vi "Fault Handling.vi"(8 "error in":errorcluster, 10 "FaultCode":i32, 11 "PostUUT in":refnum<class "PostUUT.lvclass">) -> (0 "error out":errorcluster, 3 "PostUUT out":refnum<class "PostUUT.lvclass">)   [LabVIEW 2021, in "PostUUT.lvclass"]
uses:
  PostUUT.lvclass
  PostUUT.lvclass/PostUUT.ctl
  OPC UA/OPC UA.lvclass
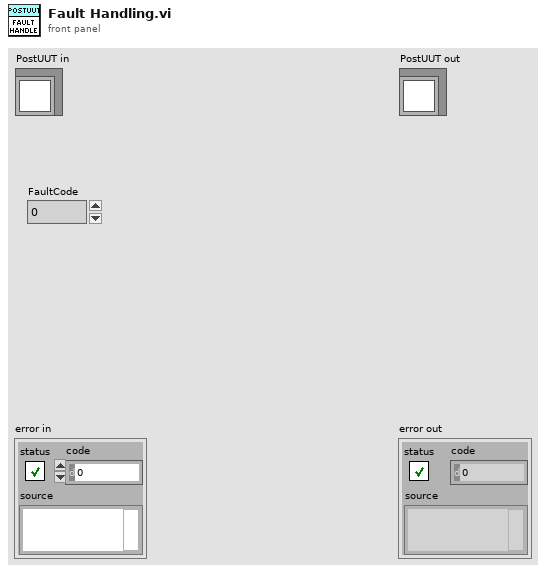
[diagram p1: front panel]
types:
  T1 = typedef "PostUUT.lvclass/Rx PostUUT.ctl" = cluster{"ResultsAck":bool, "Reset":bool, "Stop":bool, "FaultCode":u32}
  T2 = typedef "PostUUT.lvclass/Tx PostUUT.ctl" = cluster{"ResultsReady":bool, "Results":i32, "ElapsedTime":i32, "TimeCompleted":i32[], "Fault":bool, "Timeout":bool}
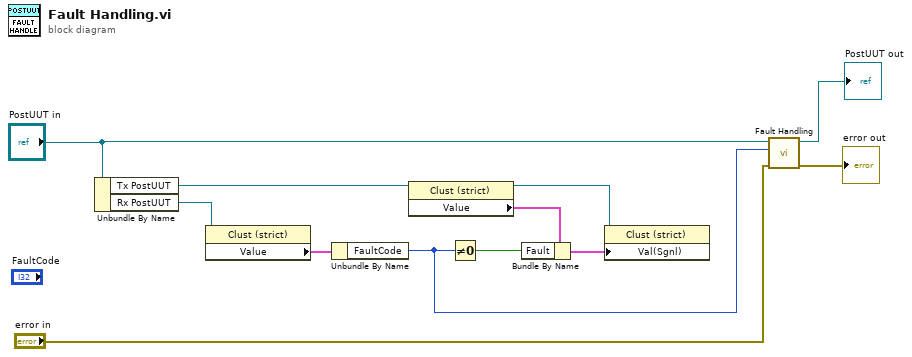
[diagram p0: block diagram]
diagram:
  n1 = Unbundle By Name("PostUUT in") -> ("Tx PostUUT"=w7:refnum<vi>, "Rx PostUUT"=w5:refnum<vi>)
  n2 = property class="Clust (strict)"(reference=w5) -> ("Value"=w6:T1)  [unwired: 1 in, 2 out]
  n3 = Unbundle By Name(w6) -> ("FaultCode"=w3:u32)
  n4 = property class="Clust (strict)"(reference=w7) -> (reference out=w10:refnum<vi>, "Value"=w8:T2)  [unwired: 1 in, 1 out]
  n5 = Not Equal To 0?(x=w3) -> (x != 0?=w2:bool)
  n6 = Bundle By Name(cluster=w8, "Fault"=w2) -> (w9:T2)
  n7 = property class="Clust (strict)"(reference=w10, "Val(Sgnl)"=w9) -> ()  [unwired: 1 in, 2 out]
  n8 = call-parent "Fault Handling.vi"("error in (no error)"="error in", "FaultCode"=w3, "OPC UA in"="PostUUT in") -> ("error out"=→"error out":errorcluster, "OPC UA out"=→"PostUUT out":refnum<class "PostUUT.lvclass">)  [unwired: 7 in]
